vi "Configure Coupling.vi"(8 "error in (no error)":errorcluster, 9 "Vertical Coupling (0: A1M)":u16(ring) items=["A1M", "A50", "D1M", "D50", "GND"], 10 "Channel (1: Channel 1)":u16(ring)=1 items=["Channel 1"=1, "Channel 2"=2, "Channel 3"=3, "Channel 4"=4], 11 "VISA resource name":refnum<visa-resource-name>) -> (0 "error out":errorcluster, 3 "VISA resource name out":refnum<visa-resource-name>)   [LabVIEW 2021, in "Siglent SDS 1000 2000 Series.lvlib"]
doc: "Specifies how you want the oscilloscope to couple the input signal for the channel."
uses:
  <instrlib>/Siglent SDS 1000 2000 Series/Siglent SDS 1000 2000 Series.lvlib
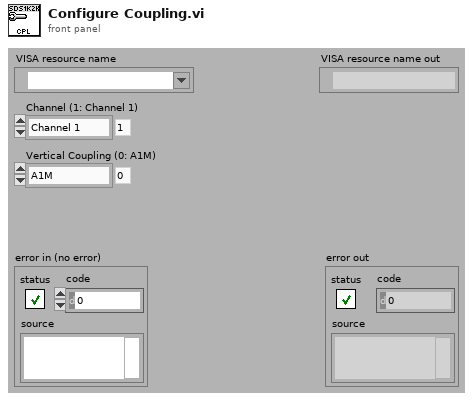
[diagram p1: front panel]
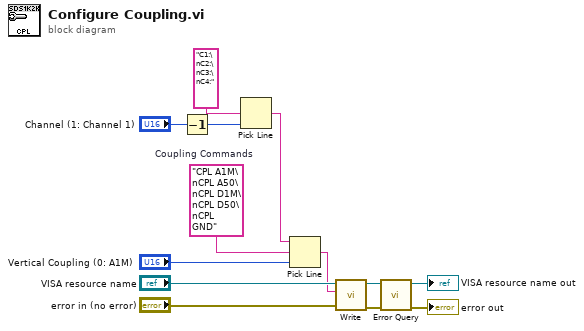
[diagram p0: block diagram]
diagram:
  w13 = "CPL A1M\nCPL A50\nCPL D1M\nCPL D50\nCPL GND"  # Coupling Commands
  n1 = Decrement(x="Channel (1: Channel 1)") -> (x-1=w1:u16)
  n2 = Pick Line(multi-line string="C1:\nC2:\nC3:\nC4:", line index=w1) -> (output string=w3:string)  [unwired: 1 in]
  n3 = Pick Line(string ("")=w3, multi-line string=w13, line index="Vertical Coupling (0: A1M)") -> (output string=w9:string)
  n4 = call <instrlib>:"Write.vi"("error in (no error)"="error in (no error)", "Write Buffer"=w9, "VISA resource name"="VISA resource name") -> ("error out"=w5:errorcluster, "VISA resource name out"=w6:refnum<visa-resource-name>)  [unwired: 6 in, 1 out]
  n5 = call <instrlib>:"Error Query.vi"("error in (no error)"=w5, "VISA resource name"=w6) -> ("error out"=→"error out":errorcluster, "VISA resource name out"=→"VISA resource name out":refnum<visa-resource-name>)  [unwired: 6 in, 2 out]
